vi "1.vi"() -> ()   [LabVIEW 2023]
panel:
  out "Waveform Chart":dbl(graph)
  in  "maxim":dbl
  in  "minim":dbl
  in  "Comutator":bool
  in  "stop":bool
  in  "stergere":bool
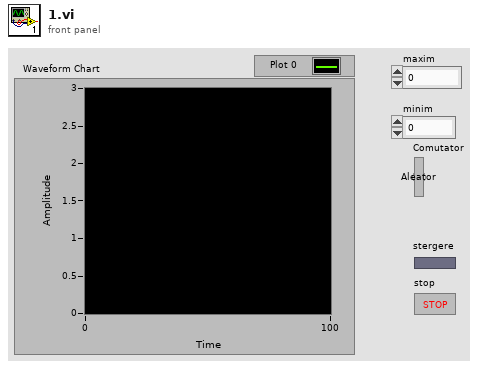
[diagram p1: front panel]
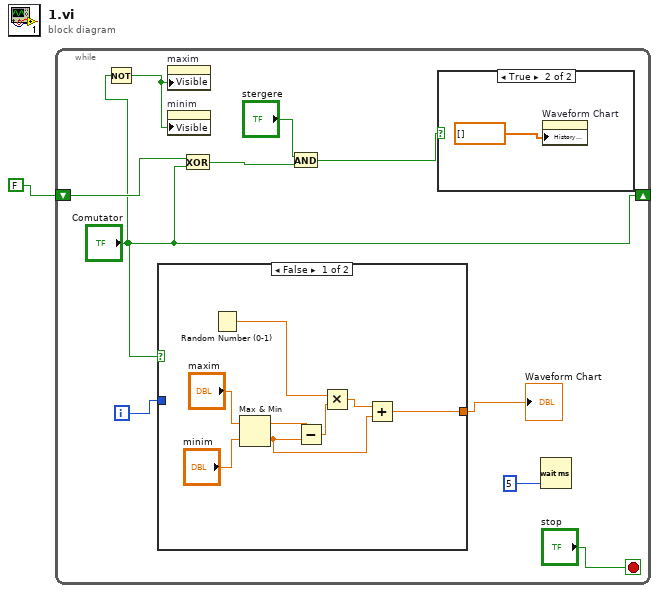
[diagram p0: block diagram]
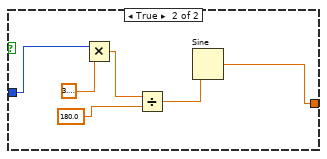
[diagram p3: hidden frame]
diagram:
  n1 = while {
    shift-right: ["Comutator"] -> _
    shift-left: FALSE -> [w6]
    i -> [w10]
    stop <- "stop" stop-if-true
    n2 = Not(x="Comutator") -> (.not. x?=w2:bool)
    n3 = case shown="False" "Comutator" {
      tunnel: w10 -> [_ w22]
      tunnel: [w13 w21] -> w3
      frame False {
        n4 = Random Number (0-1)() -> (number: 0 to 1=w20:dbl)
        n5 = Max & Min(x="maxim", y="minim") -> (max(x,y)=w15:dbl, min(x,y)=w14:dbl)
        n6 = Subtract(x=w15, y=w14) -> (x-y=w19:dbl)
        n7 = Multiply(x=w20, y=w19) -> (x*y=w18:dbl)
        n8 = Add(x=w18, y=w14) -> (x+y=w13:dbl)
      }
      frame True {
        n9 = Multiply(x=w22, y=3.141592653589793) -> (x*y=w25:dbl)
        n10 = Divide(x=w25, y=180.0) -> (x/y=w26:dbl)
        n11 = Sine(x=w26) -> (sin(x)=w21:dbl)
      }
    }
    "Waveform Chart" <- w3
    n12 = property on="maxim" class="DigNum (strict)"("Visible"=w2) -> ()  [unwired: 2 in, 2 out]
    n13 = property on="minim" class="DigNum (strict)"("Visible"=w2) -> ()  [unwired: 2 in, 2 out]
    n14 = Exclusive Or(1:"Comutator", 2:w6) -> (0:w8:bool)
    n15 = And(x="stergere", y=w8) -> (x .and. y?=w9:bool)
    n16 = case shown="True" w9 {
      frame False {
      }
      frame True {
        n17 = property on="Waveform Chart" class="WFChart (strict)"("History Data"=dbl[] []) -> ()  [unwired: 2 in, 2 out]
      }
    }
    n18 = Wait (ms)(milliseconds to wait=5) -> ()  [unwired: 1 out]
  }
